vi "LMS_UploadWFM.vi"(6 "format":i32, 7 "samples":sgl[][](array[numeric]), 8 "error in (no error)":errorcluster, 9 "sample_count":u64, 10 "ChannelCount":u8, 11 "Dev":i64) -> (0 "error out":errorcluster, 3 "Dev_out":i64)   [LabVIEW 2018, in "LMS_LV_Drv.lvlib"]
uses:
  LMS_LV_Drv.lvlib
  C:/Program Files/PothosSDR/bin/LimeSuite.dll
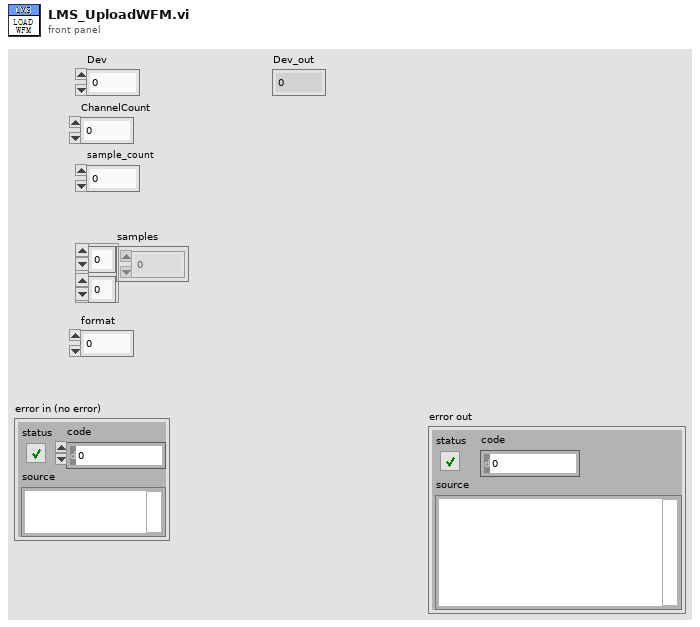
[diagram p1: front panel]
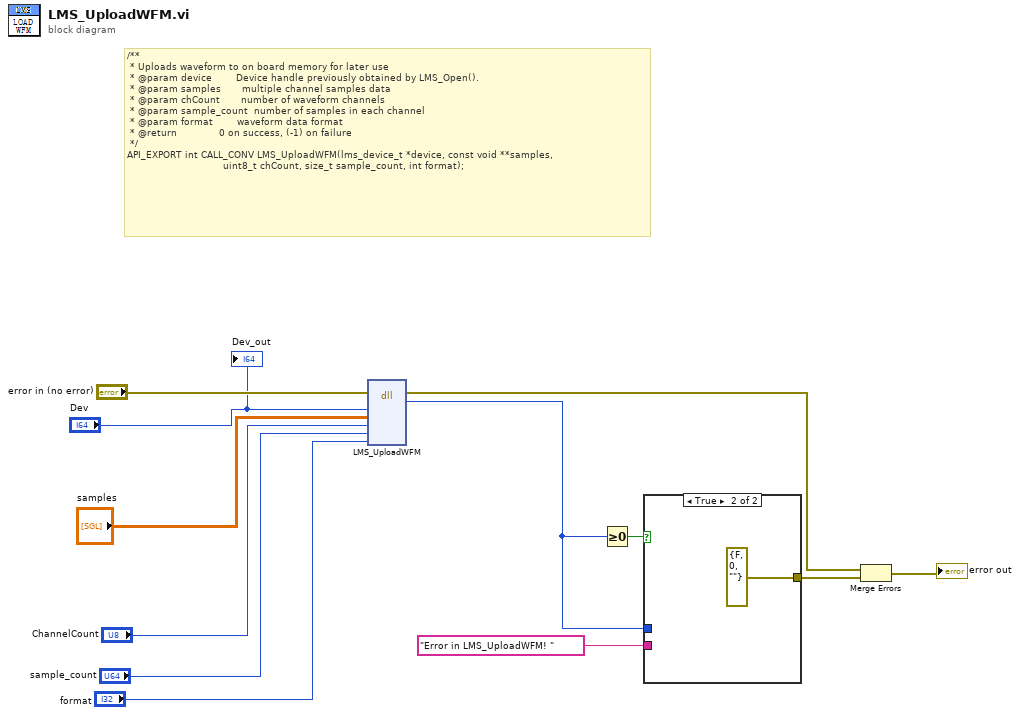
[diagram p0: block diagram]
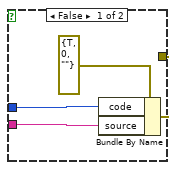
[diagram p2: hidden frame]
diagram:
  # "/**\n * Uploads waveform to on board memory for later use\n * @param device        Device handle previously obtained by LMS_Open().\n * @param samples       multiple channel samples data\n * @param chCount       number of waveform channels\n * @param sample_count  number of samples in each channel\n * @param format        waveform data format\n * @return              0 on success, (-1) on failure\n */\nAPI_EXPORT int CALL_CONV LMS_UploadWFM(lms_device_t *device, const void **samples,\n                                uint8_t chCount, size_t sample_count, int format);"
  n1 = dll-call lib="C:/Program Files/PothosSDR/bin/LimeSuite.dll" fn="LMS_UploadWFM"(error in="error in (no error)", "Dev"="Dev", "samples"="samples", "ChannelCount"="ChannelCount", "sample_count"="sample_count", "format"="format") -> (error out=w6:errorcluster, "return type"=w7:i32)  [unwired: 7 in, 1 out]
  n2 = Greater Or Equal To 0?(x=w7) -> (x >= 0?=w10:bool)
  n3 = case shown="True" w10 {
    tunnel: [w15 errorcluster {"status"=FALSE, "code"=0, "source"=""} ("error in")] -> w8
    tunnel: w7 -> [w14 _]
    tunnel: "Error in LMS_UploadWFM! " ("source") -> [w13 _]
    frame False {
      n4 = Bundle By Name(cluster=errorcluster {"status"=TRUE, "code"=0, "source"=""} ("error in"), "code"=w14, "source"=w13) -> (w15:errorcluster)
    }
    frame True {
    }
  }
  n5 = Merge Errors(w6, w8) -> (→"error out":errorcluster)
  "Dev_out" <- "Dev"
